vi "setInputGain.vi"(8 "error in (no error)":errorcluster, 10 "InputGain":dbl[](array[numeric]), 11 "Instrument.LockinAPI in":refnum<class "Instrument.LockinAPI.lvclass">) -> (0 "error out":errorcluster, 3 "Instrument.LockinAPI out":refnum<class "Instrument.LockinAPI.lvclass">)   [LabVIEW 2019, in "Instrument.LockinAPI.lvclass"]
doc: "API to put lockin into remote mode.\n\nIf address=\"\", this API reads from localhost\nIf address is remote lockin, you need to add this computer to allowed whitelist on the lockin computer you are trying to access."
uses:
  Instrument.LockinAPI.lvclass
  C:/Users/patrick/Documents/GitHub/Instrument-Framework/lvsrc/Instrument/Instrument.lvclass
  Typedefs/API/LockinAPI.Commands--Enum.ctl
  f648d4cd-a75b-428a-b411-22111a48f0ca.vi
  f648d4cd-a75b-428a-b411-22111a48f0ca.vi/d5b30f86-fbe0-4569-a0d6-a649bd9f32d7.vi
  f648d4cd-a75b-428a-b411-22111a48f0ca.vi/d5b30f86-fbe0-4569-a0d6-a649bd9f32d7.vi/3c84937f-53ed-486e-9a9e-4a7fee05ba14.vi
  f648d4cd-a75b-428a-b411-22111a48f0ca.vi/d5b30f86-fbe0-4569-a0d6-a649bd9f32d7.vi/9421ec7d-a566-4e13-98ad-1bf55e197ee0.vi
  f648d4cd-a75b-428a-b411-22111a48f0ca.vi/d5b30f86-fbe0-4569-a0d6-a649bd9f32d7.vi/c48a952f-8115-40d9-9a3e-aaed5823372a.vi
  <vilib>/JDP Science/JSONtext/Make JSON Array.vi
  f648d4cd-a75b-428a-b411-22111a48f0ca.vi/d5b30f86-fbe0-4569-a0d6-a649bd9f32d7.vi/9421ec7d-a566-4e13-98ad-1bf55e197ee0.vi/6db38ab3-4e56-4c7e-879d-311f4d7bd073.vi
  f648d4cd-a75b-428a-b411-22111a48f0ca.vi/d5b30f86-fbe0-4569-a0d6-a649bd9f32d7.vi/c48a952f-8115-40d9-9a3e-aaed5823372a.vi/5f8fc856-1fb0-4d62-ba70-aa97d4b8848d.vi
  f648d4cd-a75b-428a-b411-22111a48f0ca.vi/d5b30f86-fbe0-4569-a0d6-a649bd9f32d7.vi/c48a952f-8115-40d9-9a3e-aaed5823372a.vi/afd16ffb-2a0b-4e75-9e24-8591d20ab498.vi
  Instrument/API/Enum to String.vi
  Instrument/Private/Get RC Connection Status.vi
  <vilib>/JDP Science/JSONtext/Variant to JSON Text.vi
  <vilib>/JDP Science/JSONtext/support/Format JSON Array Text.vi
  Instrument/API/Send and Receive.vi
  <vilib>/JDP Science/JSONtext/JSON text to Variant.vi
  <vilib>/Utility/Data Type/Get Type Information.vi
  <vilib>/JDP Science/JSONtext/LVClass Serializer/JSONtext LVClass Serializer.lvclass
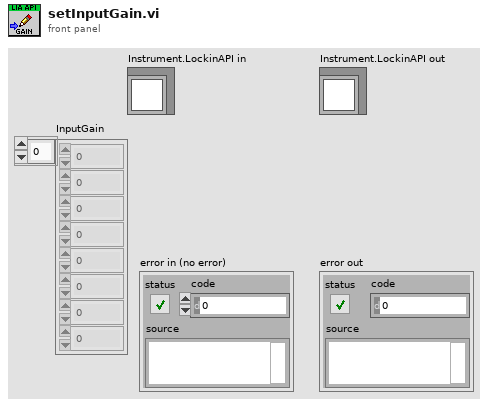
[diagram p1: front panel]
types:
  T1 = typedef "Instrument.LockinAPI.lvclass/LockinAPI.Commands--Enum.ctl" = enum16{"setAI", "setAO", "setAO_Amplitude", "setAO_DC", "setAO_Frequency", "setAO_Phase", "setAO_Function", "setAO_I+", "setREF", "setREF_Frequency", "setREF_Phase", "setREF_TC", "setREF_Roll-Off", "setDAQ", "setSampling", "setOffset", "setState", "getState", "getAO", "getAI", "getResults", "getSampling", "getAOconfig", "getREFconfig", "setInputGain", "setOutputGain", "getInputGain", "getOutputGain", "setSamplingMode", "getSamplingMode", "setSweep", "setSweepTime", "setSweepTable", "getStatus", "getSweepResults", "getSweepWaveforms", "startSweep", "stopSweep", "setAUX", "getAUX"}
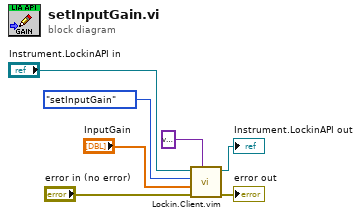
[diagram p0: block diagram]
diagram:
  n1 = call "Lockin.Client.vim"("Data Out type"=variant, "error in (no error)"="error in (no error)", "Data"="InputGain", "Command"=LockinAPI.Commands--Enum."setInputGain", "Instrument.LockinAPI in"="Instrument.LockinAPI in") -> ("error out"=→"error out":errorcluster, "Instrument.LockinAPI out"=→"Instrument.LockinAPI out":refnum<class "Instrument.LockinAPI.lvclass">)  [unwired: 4 in, 1 out]
